vi "MdsCreatePulse.vi"(2 "FlowControlIn":i32, 3 "Shot Number":i32) -> (0 "FlowControlOut":i32)   [LabVIEW 2011]
doc: "This VI will wait for an MDSplus event to occur. Currently supported when connected to an OpenVMS MDSplus data server.\n\nInputs:\n\n Event - String (required)\n FlowControlIn - Int32 (optional)\n\nOutputs:\n\n EventData - 12-byte unsigned 8-bit array (optional)\n FlowControlOut - Int32 (optional)"
panel:
  out "Status":i32
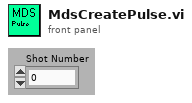
[diagram p1: front panel]
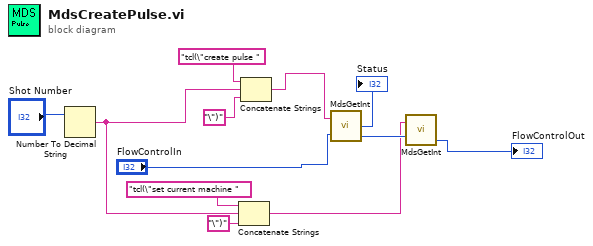
[diagram p0: block diagram]
diagram:
  n1 = Number To Decimal String(number="Shot Number") -> (decimal integer string=w3:string)  [unwired: 1 in]
  n2 = Concatenate Strings("tcl(\"set current machine " ("string"), w3, "\")" ("string")) -> (w1:string)
  n3 = Concatenate Strings("tcl(\"create pulse ", w3, "\")") -> (w9:string)
  n4 = call "MdsGetInt.vi"("Expression"=w9, "FlowControlIn"="FlowControlIn") -> ("Status"=→"Status":i32, "FlowControlOut"=w6:i32)  [unwired: 1 out]
  n5 = call "MdsGetInt.vi"("Expression"=w1, "FlowControlIn"=w6) -> ("FlowControlOut"=→"FlowControlOut":i32)  [unwired: 2 out]
